vi "yokogawa file save to usb-loop.vi"() -> ()   [LabVIEW 2011]
panel:
  in  "Seconds to wait":u32=10
  in  "stop":bool
  out "Numeric":i32
  in  "Select Trace (0: Trace A)":u16(ring) items=["Trace D", "Trace B", "Trace C", "Trace D", "Trace E", "Trace F", "Trace G"]
  out "Error Out":errorcluster
  in  "File Name (empty)":string="20150311-#8-fiber-#1"
  in  "Error In":errorcluster
  in  "VISA session":refnum<visa-resource-name>="GPIB0::1::INSTR"
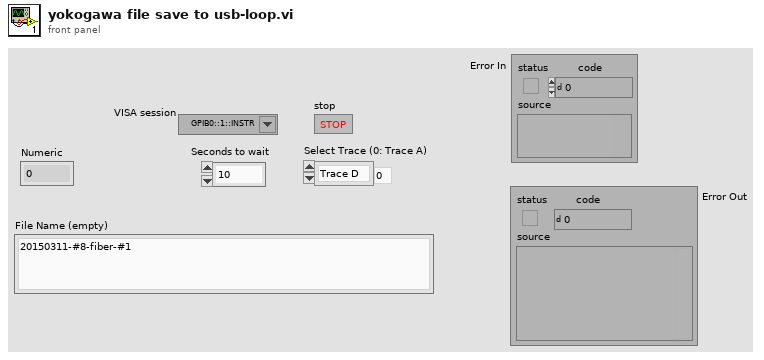
[diagram p1: front panel]
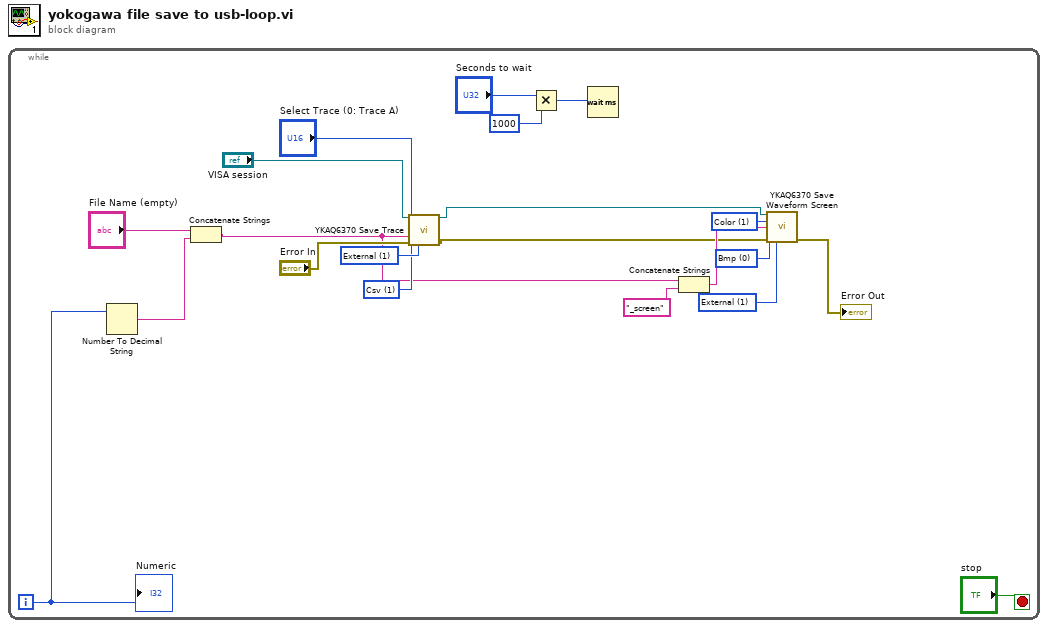
[diagram p0: block diagram]
diagram:
  n1 = while {
    i -> [w7]
    stop <- "stop" stop-if-true
    w10 = u16 1 items=["Bin", "Csv"] ("File Type (0: Bin)")
    w11 = u16 1 items=["Internal", "External"] ("Current Drive (0: Internal)")
    w12 = u16 1 items=["Internal", "External"] ("Current Drive (0: Internal)")
    w15 = u16 0 items=["Bmp", "Tiff"] ("File Type (0: Bmp)")
    w16 = u16 1 items=["B&W", "Color"] ("Color Mode (1: Color)")
    n2 = Number To Decimal String(number=w7) -> (decimal integer string=w6:string)  [unwired: 1 in]
    n3 = Concatenate Strings("File Name (empty)", w6) -> (w5:string)
    n4 = call <instrlib>:"YKAQ6370 Save Trace.vi"("VISA resource name"="VISA session", "Select Trace (0: Trace A)"="Select Trace (0: Trace A)", "File Type (0: Bin)"=w10, "File Name (empty)"=w5, "error in (no error)"="Error In", "Current Drive (0: Internal)"=w12) -> ("VISA resource name out"=w13:refnum<visa-resource-name>, "error out"=w14:errorcluster)  [unwired: 8 in]
    n5 = Multiply(x="Seconds to wait", y=u32 1000) -> (x*y=w1:u32)
    n6 = Wait (ms)(milliseconds to wait=w1) -> ()  [unwired: 1 out]
    n7 = Concatenate Strings(w5, "_screen" ("string")) -> (w17:string)
    n8 = call <instrlib>:"YKAQ6370 Save Waveform Screen.vi"("VISA resource name"=w13, "Color Mode (1: Color)"=w16, "File Name (empty)"=w17, "File Type (0: Bmp)"=w15, "error in (no error)"=w14, "Current Drive (0: Internal)"=w11) -> ("error out"=→"Error Out":errorcluster)  [unwired: 8 in, 1 out]
    "Numeric" <- w7
  }
